vi "Read Data.vi"(8 "error in (no error)":errorcluster, 11 "Tool Funnel in":refnum<class "Tool Funnel.lvclass">) -> (0 "error out":errorcluster, 2 "Path.lvclass":refnum<class "Path.lvclass">, 3 "Tool Funnel out":refnum<class "Tool Funnel.lvclass">)   [LabVIEW 2019]
uses:
  Tool Funnel.lvclass
  Parse/ParsePaths/Path.lvclass
  Tool Funnel.lvclass/Tool Funnel.ctl
  C:/Users/Albro/Documents/GitHub/AFM-Lithography/lvsrc/Classes/Tool/Tool Path/Tool Path.lvclass
  C:/Users/Albro/Documents/GitHub/AFM-Lithography/lvsrc/Classes/Tool/Tool Object/Tool Object.lvclass
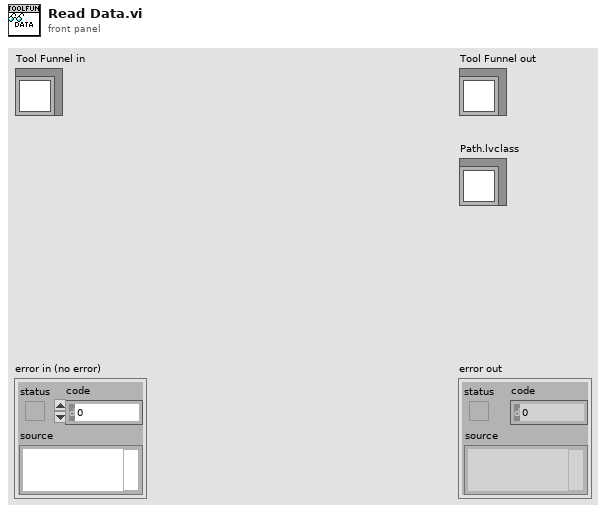
[diagram p1: front panel]
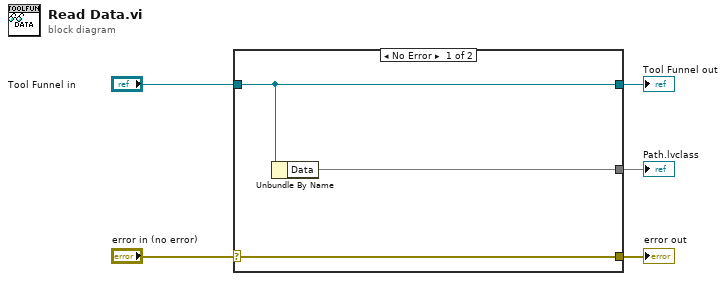
[diagram p0: block diagram]
diagram:
  n1 = case shown="No Error" "error in (no error)" {
    selector: "error in (no error)" -> [w8 w9]
    tunnel: [w8 w9] -> w4
    tunnel: [w7 w10] -> w2
    tunnel: "Tool Funnel in" -> [w7 w10]
    tunnel: [w6 _] -> w1
    frame No Error {
      n2 = Unbundle By Name(w7) -> ("Data"=w6)
    }
    frame Error {
    }
  }
  "error out" <- w4
  "Tool Funnel out" <- w2
  "Path.lvclass" <- w1
